vi "sv_Prepare Data for Resampling (Angle to Time).vi"(11 "Array":waveform(dbl)[](array[waveform])) -> (0 "channel count":i32, 1 "signal len":i32, 2 "fs":dbl format="%.2f", 3 "Y":dbl[](array[numeric]) format="%.2f", 5 "elapsed length":dbl)   [LabVIEW 2017, in "SoundVib_ContSweptSine.lvlib"]
uses:
  <vilib>/addons/Sound and Vibration/svt_Continuous Swept Sine/SoundVib_ContSweptSine.lvlib
  <vilib>/Waveform/WDTOps.llb/WDT Number of Waveform Samples DBL.vi
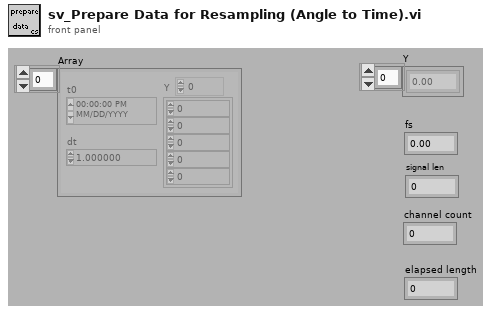
[diagram p1: front panel]
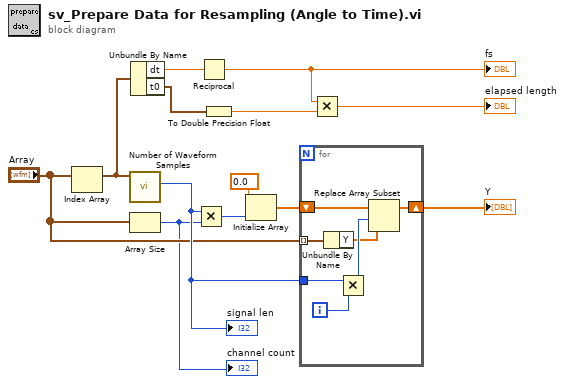
[diagram p0: block diagram]
diagram:
  n1 = Index Array(array="Array") -> (element=w5:waveform(dbl))  [unwired: 1 in]
  n2 = call-poly <vilib>:"Number of Waveform Samples.vi"("waveform in"=w5) -> ("number of samples"=w10:i32)  [unwired: 8 in, 2 out]
  "signal len" <- w10
  n3 = Array Size(array="Array") -> (size(s)=w6:i32)
  "channel count" <- w6
  n4 = Unbundle By Name(w5) -> ("dt"=w7:dbl, "t0"=w2:timestamp)
  n5 = Multiply(x=w10, y=w6) -> (x*y=w13:i32)
  n6 = Reciprocal(x=w7) -> (1/x=w3:dbl)
  "fs" <- w3
  n7 = To Double Precision Float(number=w2) -> (double precision float=w1:dbl)
  n8 = Initialize Array(0.0 ("element"), w13) -> (w11:dbl[])
  n9 = for {
    shift-right: [w14] -> w8
    shift-left: w11 -> [w20]
    tunnel: w10 -> [w18]
    tunnel: "Array" -> [w16] mode=indexing
    i -> [w19]
    n10 = Unbundle By Name(w16) -> ("Y"=w15:dbl[])
    n11 = Multiply(x=w18, y=w19) -> (x*y=w17:i32)
    n12 = Replace Array Subset(array=w20, new element=w15, index=w17) -> (w14:dbl[])
  }
  "Y" <- w8
  n13 = Multiply(x=w3, y=w1) -> (x*y=→"elapsed length":dbl)
